vi "Renishaw-XL80_Init.vi"(8 "error in (no error)":errorcluster, 11 "Renishaw-XL80_EMU in":refnum<class "Renishaw-XL80_EMU.lvclass">) -> (0 "error out":errorcluster, 1 "Serial Number":string, 2 "Connect":bool, 3 "Renishaw-XL80_EMU out":refnum<class "Renishaw-XL80_EMU.lvclass">)   [LabVIEW 2024, in "Renishaw-XL80_EMU.lvclass"]
doc: "This method connects a client to a laser measurement system.\n\nDefinition\nHRESULTConnect( [in, out] BSTR* pbstrSerNum, [out, retval] VARIANT_BOOL* pOk);\nParameters\npbstrSerNum\nDepending on your application this parameter can be used in several ways. On entry it can be set to the serial number of a specific XL laser or DX10 device to connect. It can also be blank, in which case we connect to the first available XL laser, if no laser is available we connect to the first available DX10, finally if there is no DX10 present we will connect to the first available XC weatherstation. Alternatively this can be used as a connection string to associate a specific XL laser with a specific XC compensator device, using the format \"XL:xxxxxx,XC:xxxxxx\" where xxxxxx are the serial number of each device. On return this is set to either the serial number of the DX10 which is connected, or the qualified string for the connected laser system e.g. \"XL:xxxxxx,XC:xxxxxx \"\n\npOk\nA variable that will be set to VARIANT_TRUE or VARIANT_FALSE. If the variable is set to VARIANT_TRUE then the client has successfully connected to either a XL laser or DX10 device.\n\nComments\nThis method should be called before any other property or method. Most of the other methods supported by this interface will return E_FAIL if the client has not already connected. The client should keep trying to connect until it succeeds.\n\nThe method will usually return a HRESULT of S_OK. However, it will return E_POINTER if the client supplies null pointers for either pOk or pbstrSerNum, and in extremely low memory conditions it will return E_NOMEMORY.\n\nThe method may fail to connect a client to a laser system under any of the following conditions:\n\nthe client specified a XL laser system or DX10 that is not attached to the PC \nthere are no XL lasers, DX10s, or XC weatherstations attached to the PC \nall XL laser systems and DX10s attached to the PC are connected to other clients. \nNote that if the client has already connected to either a XL laser or DX10 then this method will succeed. It will set pOk to VARIANT_TRUE and set pbstrSerNum to the serial number or qualified string of the connected devices.\n\nIf this method successfully connects to a XL laser we return a pOk of VARIANT_TRUE regardless of the XC compensator's connection status. We will continue to poll the XC for connection and return a status of EC10_NOT_RESPONDING. If the XC's serial number is not specified as in the connection string above, any available XC will be connected and associated with the XL laser.\n\nIf this method successfully connects to a XC weatherstation we return a pOk of VARIANT_TRUE regardless of the XL laser's connection status. We will continue to poll the XL for connection and return a status of ML10_NOT_RESPONDING. If the XL's serial number is not specified as in the connection string above, any available XL will be connected and associated with the XC weatherstation. \n\nIt is important that the client application calls Disconnect before it exits. For most languages this will be done automatically when the last reference to the COM object is released, but we have found some, notably C#, that wait until garbage collection to release the COM object. Garbage collection may occur at any time. This can mean that the DX10 remains unavailable to other clients.\n\nA similar effect may occur if the client crashes before calling Disconnect. In both cases, if you are connected to a DX10, restarting DX10Server.exe is the only way to recover."
uses:
  Renishaw-XL80_EMU.lvclass
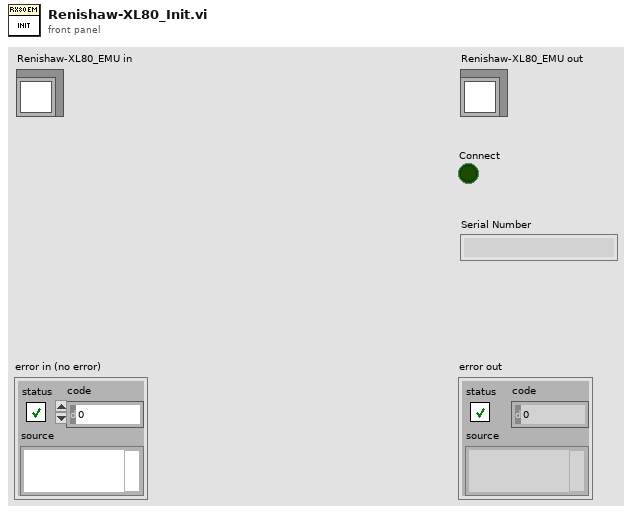
[diagram p1: front panel]
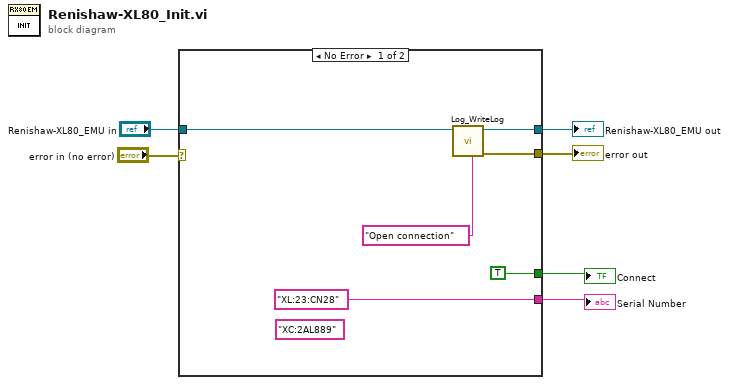
[diagram p0: block diagram]
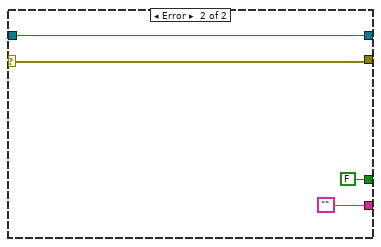
[diagram p2: hidden frame]
diagram:
  n1 = case shown="No Error" "error in (no error)" {
    selector: "error in (no error)" -> [_ w15]
    tunnel: "Renishaw-XL80_EMU in" -> [w11 w16]
    tunnel: [w10 w16] -> w5
    tunnel: [w9 w15] -> w3
    tunnel: [TRUE ("Connect") FALSE ("Connect")] -> w2
    tunnel: ["XL:23:CN28" ("Serial Number") ""] -> w1
    frame No Error {
      (unwired) "XC:2AL889" ("Serial Number")
      n2 = call-dynamic "Log_WriteLog.vi"("Additional text"="Open connection", "Log in"=w11) -> ("error out"=w9:errorcluster, "Log out"=w10:refnum<class "Renishaw-XL80_EMU.lvclass">)  [unwired: 8 in]
    }
    frame Error {
    }
  }
  "error out" <- w3
  "Renishaw-XL80_EMU out" <- w5
  "Connect" <- w2
  "Serial Number" <- w1
